vi "DisableEnable.vi"(8 "error in (no error)":errorcluster, 9 "Action 2":T1=enum." Grayed Out", 11 "Array of Control References":refnum<vi>[](array[refnum])) -> (0 "error out":errorcluster)   [LabVIEW 2012]
uses:
  type def/Hyde&Show.ctl
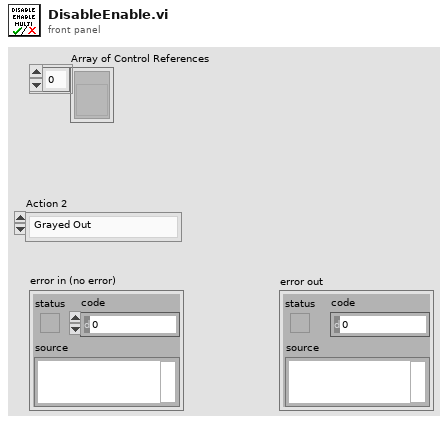
[diagram p1: front panel]
types:
  T1 = typedef "Hyde&Show.ctl" = enum8{"Enabled", "Disabled", " Grayed Out", "Hide"}
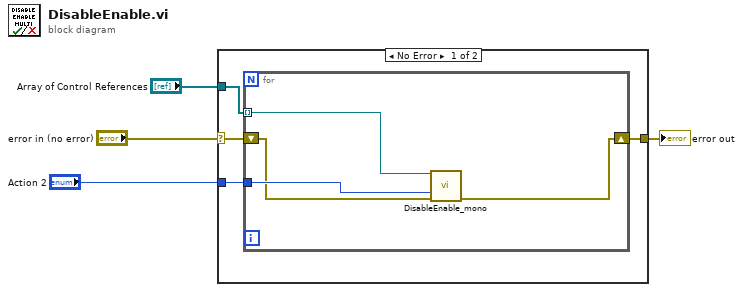
[diagram p0: block diagram]
diagram:
  n1 = case shown="No Error" "error in (no error)" {
    selector: "error in (no error)" -> [w6 w13]
    tunnel: "Action 2" -> [w7 _]
    tunnel: "Array of Control References" -> [w5 _]
    tunnel: [w8 w13] -> w1
    frame No Error {
      n2 = for {
        tunnel: w5 -> [w12] mode=indexing
        shift-right: [w9] -> w8
        shift-left: w6 -> [w10]
        tunnel: w7 -> [w11]
        n3 = call "DisableEnable_mono.vi"("Control in"=w12, "Action in"=w11, "error in (no error)"=w10) -> ("error out"=w9:errorcluster)  [unwired: 12 in]
      }
    }
    frame Error {
    }
  }
  "error out" <- w1
